vi "Application Path AE.vi"(10 "Application Path in":path) -> (2 "Application Path out":path)   [LabVIEW 2025]
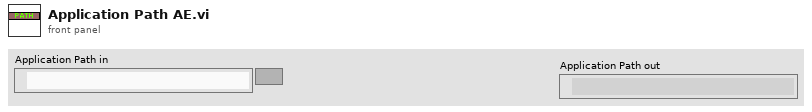
[diagram p1: front panel]
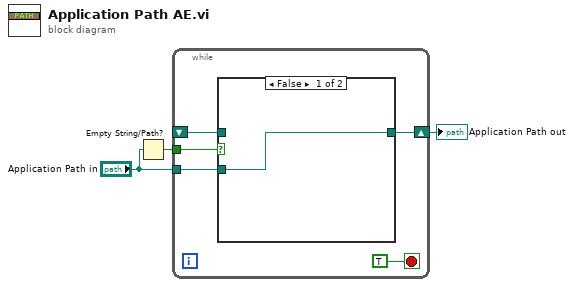
[diagram p0: block diagram]
diagram:
  n1 = Empty String/Path?(string/path="Application Path in") -> (empty?=w2:bool)
  n2 = while {
    tunnel: "Application Path in" -> [w8]
    tunnel: w2 -> [w7]
    shift-right: [w6] -> w1
    shift-left: _ -> [w5]
    stop <- TRUE stop-if-true
    n3 = case shown="False" w7 {
      tunnel: w8 -> [w9 _]
      tunnel: [w9 w10] -> w6
      tunnel: w5 -> [_ w10]
      frame False {
      }
      frame True {
      }
    }
  }
  "Application Path out" <- w1
